vi "Server_command_head_nod.vi"() -> ()   [LabVIEW 2013]
doc: "Template server that runs individual ros topics, services, etc. This is cloned for each topic being run."
uses:
  ROS/Code/SubVIs/_ROSControl.ctl
  ROS/Code/SubVIs/_ROSDirection.ctl
panel:
  in  "queue":string="/robot/head/command_head_nodQueue"
  out "Connected":bool=TRUE
  out "Status":T1(ring) caption="Connected?"
  out "Specs":T3={"Server"="/robot/head/command_head_nod", "Node"="/labview", "Server Port"=59814, "URI (Subsc)"="192.168.0.11:52023", "Direction"=enum."Publisher"}
  in  "stop":bool
  out "error out":errorcluster
  out "Connections":T4(array[cluster])=[{"Caller ID"="/realtime_loop", "Topic Name"="/robot/head/command_head_nod", "Protocol"="TCPROS", "URIs"="192.168.0.11:52023"}]
  in  "Baxter":T5={"topic port"=59814, "Node"="/labview", "topic"="/robot/head/command_head_nod", "type"="std_msgs/Bool", "node port"=7000, "error "={"status"=FALSE, "code"=0, "source"=""}, "Direction"=enum."Publisher", "APIs"=[]}
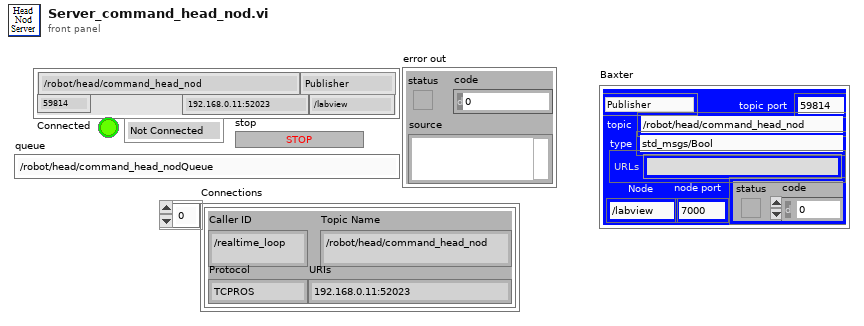
[diagram p1: front panel]
types:
  T1 = enum16{"Not Connected", "Registered", "Connected"}
  T2 = typedef "_ROSDirection.ctl" = enum16{"Node", "Publisher", "Subscriber", "Service Client"}
  T3 = cluster{"Server":string, "Node":string, "Server Port":u32, "URI (Subsc)":string, "Direction":T2}
  T4 = cluster{"Caller ID":string, "Topic Name":string, "Protocol":string, "URIs":string}[]
  T5 = typedef "_ROSControl.ctl" = cluster{"topic port":u16, "Node":string, "topic":string, "type":string, "node port":u32, "error ":errorcluster, "Direction":T2, "APIs":string[]}
  T6 = cluster{"Caller ID":string, "Topic Name":string, "Protocol":string, "URIs":string}
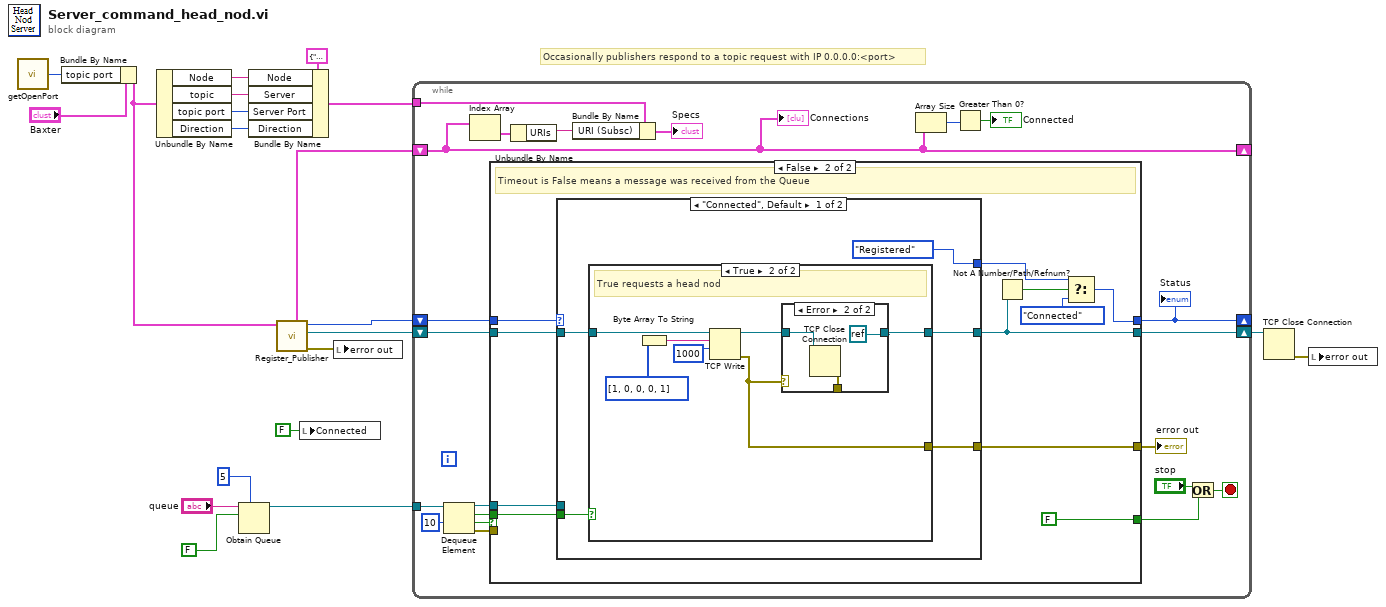
[diagram p0: block diagram]
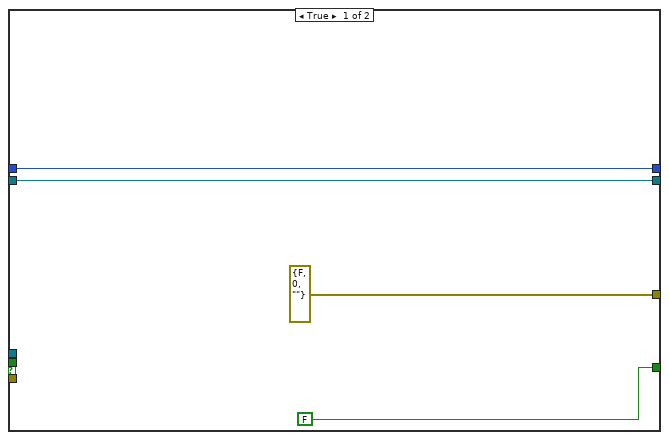
[diagram p2: hidden frame]
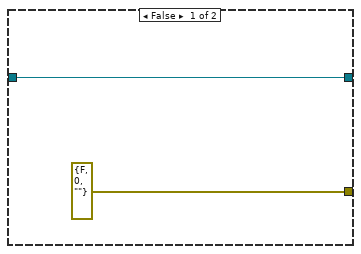
[diagram p3: hidden frame]
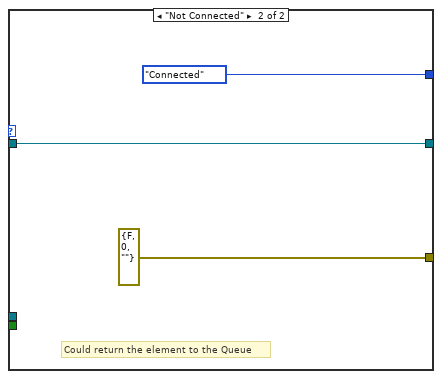
[diagram p5: hidden frame]
diagram:
  # "Occasionally publishers respond to a topic request with IP 0.0.0.0:<port>"
  n1 = call "getOpenPort.vi"() -> ("port"=w6:u16)
  n2 = Bundle By Name(cluster="Baxter", "topic port"=w6) -> (w5:T5)
  n3 = Unbundle By Name(w5) -> ("Node"=w18:string, "topic"=w17:string, "topic port"=w15:u16, "Direction"=w16:T2)
  n4 = Obtain Queue(max queue size (-1, unlimited)=5, name (unnamed)="queue", element data type=FALSE) -> (queue out=w11:refnum<queue>)  [unwired: 2 in, 2 out]
  n5 = Bundle By Name(cluster=T3 {"Server"="", "Node"="/labview", "Server Port"=5000, "URI (Subsc)"="", "Direction"=enum."Node"} ("Specs"), "Node"=w18, "Server"=w17, "Server Port"=w15, "Direction"=w16) -> (w19:T3)
  n6 = call "Register_Publisher.vi"("Baxter"=w5) -> ("error out"=w1:errorcluster, "connection ID out"=w2:refnum<k5>, "Status"=w3:T1, "Subscribers"=w4:T4)  [unwired: 7 in]
  n7 = local write "Connected"(FALSE ("Connected")) -> ()
  n8 = local write "error out"(w1) -> ()
  n9 = while {
    shift-right: [w21] -> _
    shift-left: w4 -> [w21]
    shift-right: [w39] -> w10
    shift-left: w2 -> [w41]
    shift-right: [w37] -> _
    shift-left: w3 -> [w38]
    tunnel: w19 -> [w34]
    tunnel: w11 -> [w27]
    stop <- w22 stop-if-true
    n10 = Dequeue Element(queue=w27, timeout in ms (-1)=10) -> (queue out=w31:refnum<queue>, element=w25:bool, timed out?=w26:bool, error out=w28:errorcluster)  [unwired: 1 in]
    n11 = Index Array(array=w21) -> (element=w35:T6)  [unwired: 1 in]
    n12 = case shown="False" w26 {
      tunnel: [w45 w53] -> w39
      tunnel: w41 -> [w45 w56]
      tunnel: [FALSE FALSE] -> w23
      tunnel: [errorcluster {"status"=FALSE, "code"=0, "source"=""} ("error out") w54] -> w36
      tunnel: w38 -> [w44 w55]
      tunnel: [w44 w48] -> w37
      tunnel: w31 -> [_ w52]
      tunnel: w28 -> [_ _]
      tunnel: w25 -> [_ w46]
      frame True {
      }
      frame False {
        # "Timeout is False means a message was received from the Queue"
        n13 = case shown="\"Connected\", Default" w55 {
          tunnel: w56 -> [w61 w77]
          tunnel: [w59 w77] -> w53
          tunnel: [w60 errorcluster {"status"=FALSE, "code"=0, "source"=""} ("error out")] -> w54
          tunnel: w52 -> [_ _]
          tunnel: [T1."Registered" ("f") T1."Connected" ("f")] -> w49
          tunnel: w46 -> [w57 _]
          frame "Connected", Default {
            n14 = case shown="True" w57 {
              tunnel: w61 -> [w62 w70]
              tunnel: [errorcluster {"status"=FALSE, "code"=0, "source"=""} ("error out") w69] -> w60
              tunnel: [w62 w68] -> w59
              frame False {
              }
              frame True {
                # "True requests a head nod"
                n15 = Byte Array To String(unsigned byte array=u8[] [1, 0, 0, 0, 1]) -> (string=w64:string)
                n16 = TCP Write(connection ID=w70, data in=w64, 9:1000 ("timeout ms (25000)")) -> (connection ID out=w66:refnum<k5>, error out=w69:errorcluster)  [unwired: 1 in, 1 out]
                n17 = case shown="Error" w69 {
                  tunnel: w66 -> [w71 w74]
                  tunnel: [w71 refnum<k0> refnum] -> w68
                  tunnel: [_ w72] -> _
                  frame No Error {
                  }
                  frame Error {
                    n18 = TCP Close Connection(connection ID=w74) -> (error out=w72:errorcluster)  [unwired: 2 in, 1 out]
                  }
                }
              }
            }
          }
          frame "Not Connected" {
            # "Could return the element to the Queue"
          }
        }
        n19 = Not A Number/Path/Refnum?(number/path/refnum=w53) -> (NaN/Path/Refnum?=w50:bool)
        n20 = Select(t=w49, s=w50, f=T1."Connected") -> (s? t:f=w48:T1)
      }
    }
    "error out" <- w36
    "Status" <- w37
    n21 = Unbundle By Name(w35) -> ("URIs"=w33:string)
    n22 = Bundle By Name(cluster=w34, "URI (Subsc)"=w33) -> (→"Specs":T3)
    n23 = Array Size(array=w21) -> (size(s)=w30:i32)
    n24 = Greater Than 0?(x=w30) -> (x > 0?=→"Connected":bool)
    n25 = Or(x="stop", y=w23) -> (x .or. y?=w22:bool)
    "Connections" <- w21
  }
  n26 = TCP Close Connection(connection ID=w10) -> (error out=w9:errorcluster)  [unwired: 2 in, 1 out]
  n27 = local write "error out"(w9) -> ()
